vi "TMCM351-STOP.vi"(2 "错误输入":errorcluster caption="错误输入（无错误）", 3 "motor":u8(ring) items=["x", "y", "z"], 4 "com in":refnum<visa-resource-name>) -> (0 "错误输出":errorcluster, 1 "com out":refnum<visa-resource-name>)   [LabVIEW 2018]
uses:
  module_param.vi
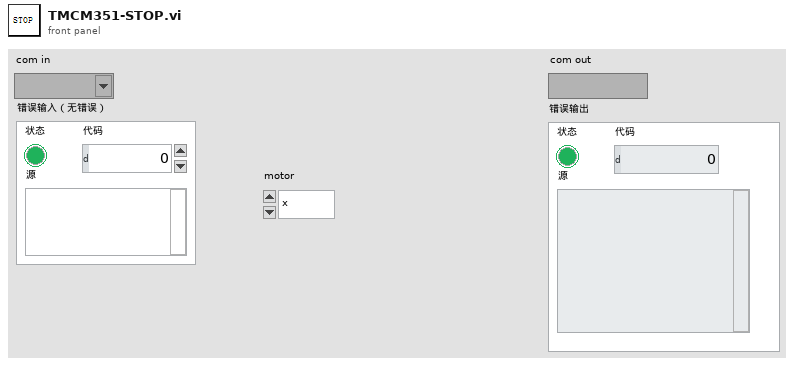
[diagram p1: front panel]
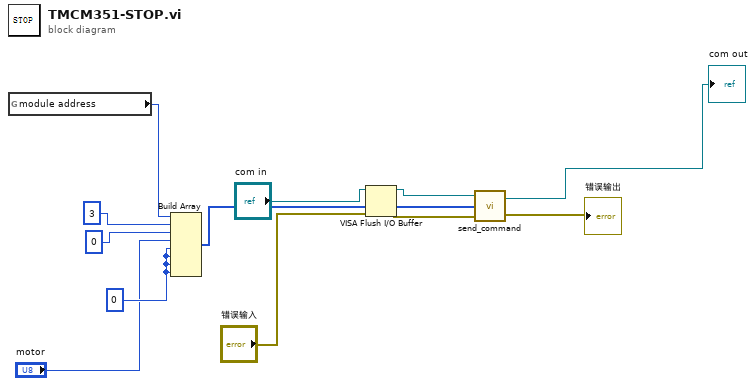
[diagram p0: block diagram]
diagram:
  w10 = u8 0 ("元素")
  n1 = global read "module_param.vi" "module address"() -> (w9:u8)
  n2 = Build Array(w9, u8 3, u8 0, "motor", w10, w10, w10, w10) -> (w7:u8[])
  n3 = VISA Flush I/O Buffer(VISA resource name="com in", error in (no error)="错误输入") -> (VISA resource name out=w4:refnum<visa-resource-name>, error out=w3:errorcluster)  [unwired: 1 in]
  n4 = call "send_command.vi"("错误输入"=w3, 3:w7, "com in"=w4) -> ("错误输出"=→"错误输出":errorcluster, "com out"=→"com out":refnum<visa-resource-name>)
